vi "Configure Limit Test Stop After.vi"(6 "Waveform (0.0)":dbl, 7 "Time (0.0 s)":dbl, 8 "error in (no error)":errorcluster, 9 "Violation (0.0)":dbl, 10 "Mode (0:Channel 1)":i32(ring) items=["Manual", "Waveform", "Violation", "Time"], 11 "VISA resource name":refnum<visa-resource-name>) -> (0 "error out":errorcluster, 3 "VISA resource name out":refnum<visa-resource-name>)   [LabVIEW 2017, in "Tektronix TDS 200 1000 2000 Series.lvlib"]
doc: "This VI configures the settings for a limit test stop after.\n\n<b>Note(s):</b>\nThis VI does not check the instrument status."
uses:
  Tektronix TDS 200 1000 2000 Series.lvlib
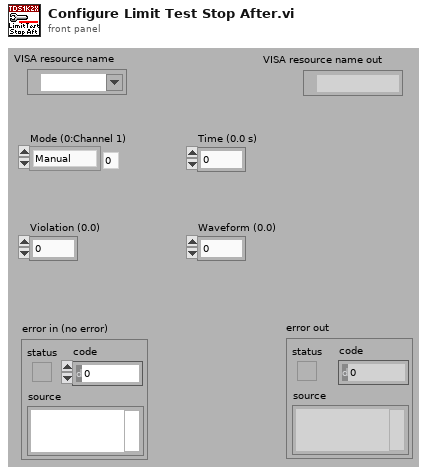
[diagram p1: front panel]
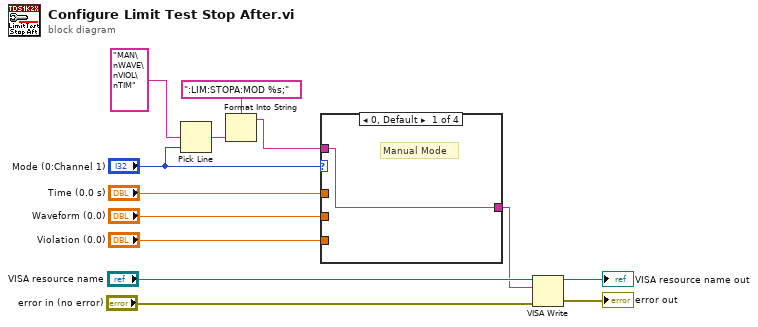
[diagram p0: block diagram]
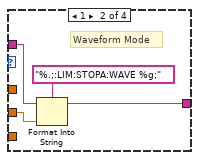
[diagram p2: hidden frame]
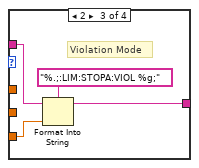
[diagram p3: hidden frame]
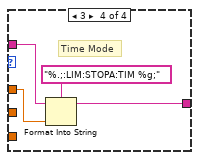
[diagram p4: hidden frame]
diagram:
  n1 = Pick Line(multi-line string="MAN\nWAVE\nVIOL\nTIM", line index="Mode (0:Channel 1)") -> (output string=w9:string)  [unwired: 1 out]
  n2 = Format Into String(format string=":LIM:STOPA:MOD %s;", w9) -> (resulting string=w5:string)  [unwired: 2 in, 1 out]
  n3 = case shown="0, Default" "Mode (0:Channel 1)" {
    tunnel: w5 -> [w14 w17 w21 w25]
    tunnel: [w14 w16 w20 w24] -> w4
    tunnel: "Waveform (0.0)" -> [_ w15 _ _]
    tunnel: "Violation (0.0)" -> [_ _ w19 _]
    tunnel: "Time (0.0 s)" -> [_ _ _ w23]
    frame 0, Default {
      # "Manual Mode"
    }
    frame 1 {
      # "Waveform Mode"
      n4 = Format Into String(format string="%.;:LIM:STOPA:WAVE %g;", initial string=w17, w15) -> (resulting string=w16:string)  [unwired: 1 in, 1 out]
    }
    frame 2 {
      # "Violation Mode"
      n5 = Format Into String(format string="%.;:LIM:STOPA:VIOL %g;", initial string=w21, w19) -> (resulting string=w20:string)  [unwired: 1 in, 1 out]
    }
    frame 3 {
      # "Time Mode"
      n6 = Format Into String(format string="%.;:LIM:STOPA:TIM %g;", initial string=w25, w23) -> (resulting string=w24:string)  [unwired: 1 in, 1 out]
    }
  }
  n7 = VISA Write(VISA resource name="VISA resource name", write buffer=w4, error in (no error)="error in (no error)") -> (VISA resource name out=→"VISA resource name out":refnum<visa-resource-name>, error out=→"error out":errorcluster)  [unwired: 1 out]
